vi "SubDataDyn.vi"(10 "cluster":T2, 11 "Cluster en entrée":T1) -> (2 "Chaîne":string, 3 "cluster de sortie":T1)   [LabVIEW 2020]
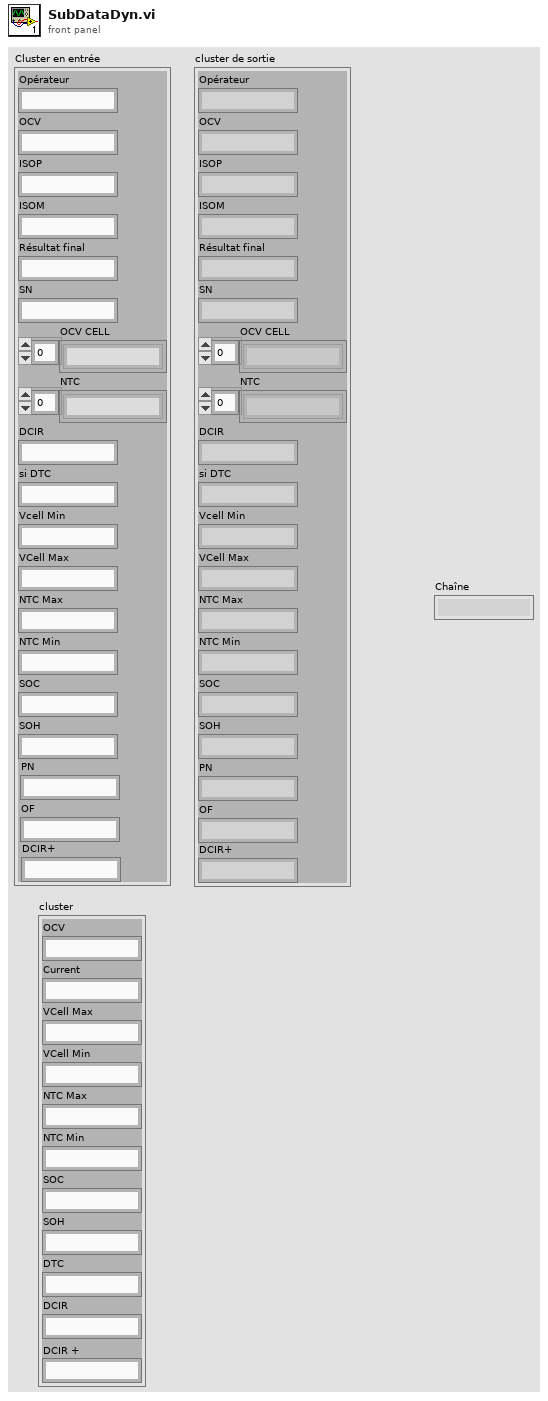
[diagram p1: front panel]
types:
  T1 = cluster{"Opérateur":string, "OCV":string, "ISOP":string, "ISOM":string, "Résultat final":string, "SN":string, "OCV CELL":string[], "NTC":string[], "DCIR":string, "si DTC":string, "Vcell Min":string, "VCell Max":string, "NTC Max":string, "NTC Min":string, "SOC":string, "SOH":string, "PN":string, "OF":string, "DCIR+":string}
  T2 = cluster{"OCV":string, "Current":string, "VCell Max":string, "VCell Min":string, "NTC Max":string, "NTC Min":string, "SOC":string, "SOH":string, "DTC":string, "DCIR":string, "DCIR +":string}
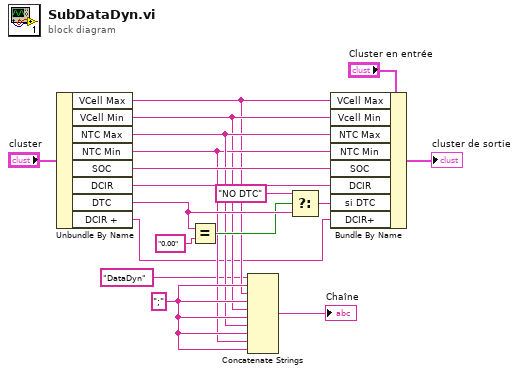
[diagram p0: block diagram]
diagram:
  w11 = ";" ("chaîne")
  n1 = Unbundle By Name("cluster") -> ("VCell Max"=w7:string, "VCell Min"=w8:string, "NTC Max"=w10:string, "NTC Min"=w9:string, "SOC"=w12:string, "DCIR"=w13:string, "DTC"=w16:string, "DCIR +"=w1:string)
  n2 = Equal?(x=w16, y="0.00") -> (x = y?=w15:bool)
  n3 = Concatenate Strings("DataDyn" ("chaîne"), w11, w7, w11, w8, w11, w10, w11, w9, w11) -> (→"Chaîne":string)
  n4 = Select(t="NO DTC" ("cas vrai"), s=w15, f=w16) -> (s? t:f=w17:string)
  n5 = Bundle By Name(cluster="Cluster en entrée", "VCell Max"=w7, "Vcell Min"=w8, "NTC Max"=w10, "NTC Min"=w9, "SOC"=w12, "DCIR"=w13, "si DTC"=w17, "DCIR+"=w1) -> (→"cluster de sortie":T1)
